vi "Check Resources (SubVI).vi"(8 "error in (no error)":errorcluster, 9 "Language":enum16{"English", "Deutsch", "Italiano"}(ring), 10 "Language Data":string[][](array[string]), 11 "Simulation":cluster{"Water":dbl, "Coffee":dbl, "Milk":dbl}) -> (0 "error out":errorcluster, 1 "Coffee ok?":bool, 2 "Milk ok?":bool, 3 "Water ok?":bool, 5 "Status Message":string)   [LabVIEW 2017]
panel:
  # "Input Values"
  # "Output Values"
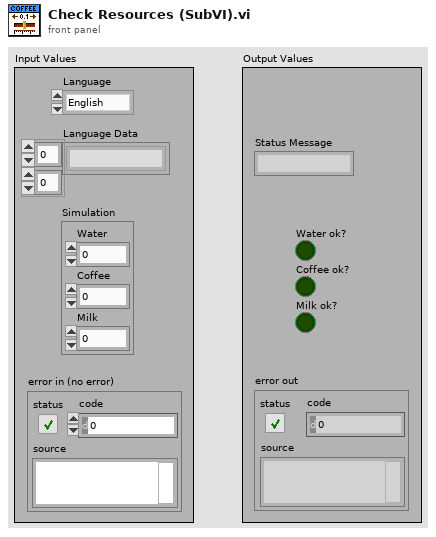
[diagram p1: front panel]
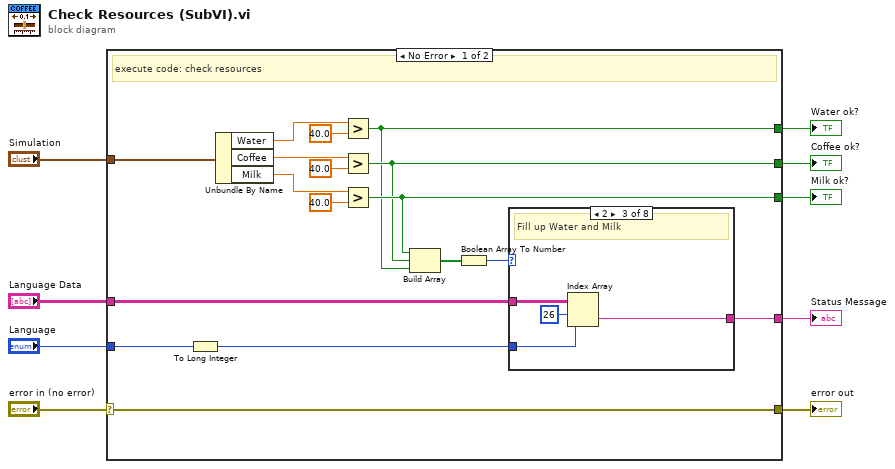
[diagram p0: block diagram]
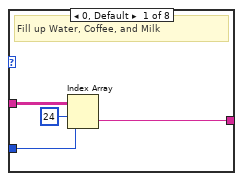
[diagram p2: hidden frame]
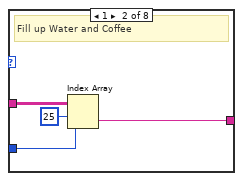
[diagram p3: hidden frame]
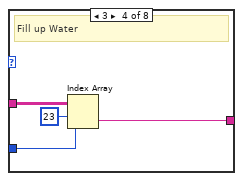
[diagram p4: hidden frame]
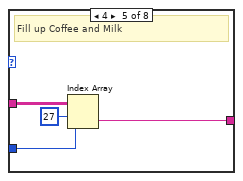
[diagram p5: hidden frame]
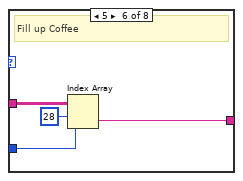
[diagram p6: hidden frame]
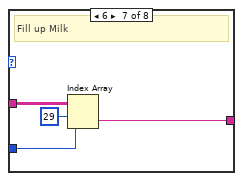
[diagram p7: hidden frame]
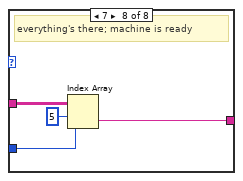
[diagram p8: hidden frame]
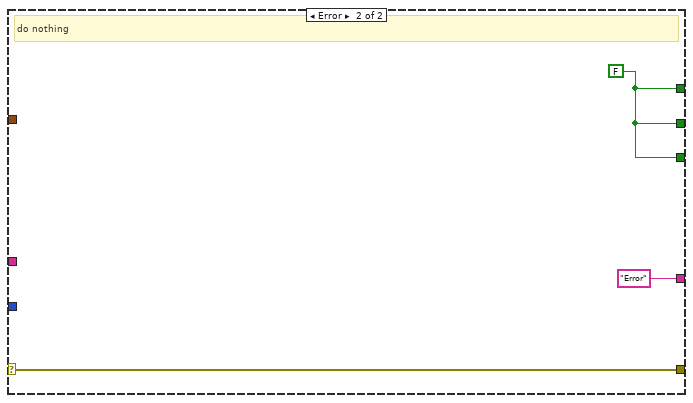
[diagram p9: hidden frame]
diagram:
  n1 = case shown="No Error" "error in (no error)" {
    selector: "error in (no error)" -> [w25 w61]
    tunnel: "Language Data" -> [w13 _]
    tunnel: "Simulation" -> [w26 _]
    tunnel: [w25 w61] -> w6
    tunnel: [w16 w60] -> w5
    tunnel: [w17 w60] -> w4
    tunnel: [w18 w60] -> w3
    tunnel: "Language" -> [w12 _]
    tunnel: [w10 "Error" ("String")] -> w1
    frame No Error {
      # "execute code: check resources"
      n2 = To Long Integer(number=w12) -> (32bit integer=w11:i32)
      n3 = Unbundle By Name(w26) -> ("Water"=w21:dbl, "Coffee"=w20:dbl, "Milk"=w19:dbl)
      n4 = Greater?(x=w21, y=40.0) -> (0:w16:bool)
      n5 = Greater?(x=w20, y=40.0) -> (0:w17:bool)
      n6 = Greater?(x=w19, y=40.0) -> (0:w18:bool)
      n7 = Build Array(w18, w17, w16) -> (w15:bool[])
      n8 = Boolean Array To Number(Boolean array=w15) -> (number=w14:u32)
      n9 = case shown="2" w14 {
        tunnel: w13 -> [w30 w34 w38 w42 w46 w50 w54 w58]
        tunnel: w11 -> [w29 w33 w37 w41 w45 w49 w53 w57]
        tunnel: [w28 w32 w36 w40 w44 w48 w52 w56] -> w10
        frame 0, Default {
          # "Fill up Water, Coffee, and Milk"
          n10 = Index Array(array=w30, index (row)=24 ("disabled index (row)"), index (col)=w29) -> (element=w28:string)
        }
        frame 1 {
          # "Fill up Water and Coffee"
          n11 = Index Array(array=w34, index (row)=25 ("disabled index (row)"), index (col)=w33) -> (element=w32:string)
        }
        frame 2 {
          # "Fill up Water and Milk"
          n12 = Index Array(array=w38, index (row)=26 ("disabled index (row)"), index (col)=w37) -> (element=w36:string)
        }
        frame 3 {
          # "Fill up Water"
          n13 = Index Array(array=w42, index (row)=23 ("disabled index (row)"), index (col)=w41) -> (element=w40:string)
        }
        frame 4 {
          # "Fill up Coffee and Milk"
          n14 = Index Array(array=w46, index (row)=27 ("disabled index (row)"), index (col)=w45) -> (element=w44:string)
        }
        frame 5 {
          # "Fill up Coffee"
          n15 = Index Array(array=w50, index (row)=28 ("disabled index (row)"), index (col)=w49) -> (element=w48:string)
        }
        frame 6 {
          # "Fill up Milk"
          n16 = Index Array(array=w54, index (row)=29 ("disabled index (row)"), index (col)=w53) -> (element=w52:string)
        }
        frame 7 {
          # "everything's there; machine is ready"
          n17 = Index Array(array=w58, index (row)=5 ("disabled index (row)"), index (col)=w57) -> (element=w56:string)
        }
      }
    }
    frame Error {
      w60 = FALSE
      # "do nothing"
    }
  }
  "error out" <- w6
  "Water ok?" <- w5
  "Coffee ok?" <- w4
  "Milk ok?" <- w3
  "Status Message" <- w1
